vi "DSF.Engine.Memory.ObjectPool.Return Object.vi"(8 "error in (no error)":errorcluster, 9 "timeout ms (0)":i32 format="%d ms", 10 "ObjectPool Bundle":refnum<class "DSF.Engine.Memory.ObjectPool.Bundle.lvclass">, 11 "ObjectPool in":refnum<class "DSF.Engine.Memory.ObjectPool.lvclass">) -> (0 "error out":errorcluster, 1 "timed out?":bool, 3 "ObjectPool out":refnum<class "DSF.Engine.Memory.ObjectPool.lvclass">)   [LabVIEW 2016, in "DSF.Engine.lvlib" / "DSF.Engine.Memory.ObjectPool.lvclass"]
uses:
  DSF.Engine.Memory.ObjectPool.lvclass
  DSF.Engine.Memory.ObjectPool.Bundle.lvclass
  DSF.Engine.Memory.ObjectPool.Bundle.lvclass/DSF.Engine.Memory.ObjectPool.Bundle.ctl
  DSF.Engine.Memory.ObjectPool.lvclass/DSF.Engine.Memory.ObjectPool.ctl
  DSF.Engine.Memory.ObjectPool.Get Index FIFO.vi
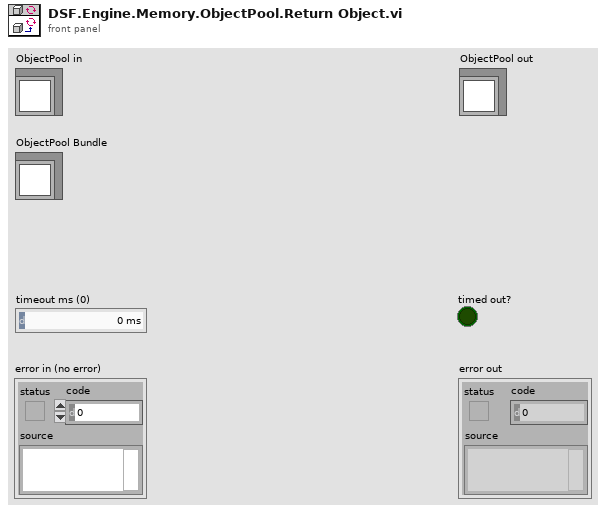
[diagram p1: front panel]
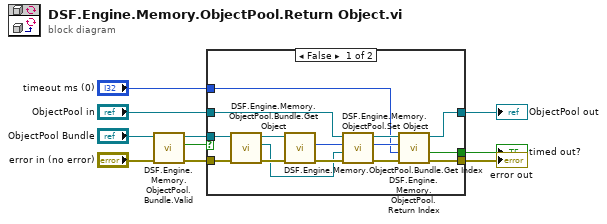
[diagram p0: block diagram]
diagram:
  n1 = call "DSF.Engine.Memory.ObjectPool.Bundle.Valid.vi"("error in (no error)"="error in (no error)", "ObjectPool Bundle in"="ObjectPool Bundle") -> ("error out"=w10:errorcluster, "valid?"=w3:bool, "ObjectPool Bundle out"=w4:refnum<class "DSF.Engine.Memory.ObjectPool.Bundle.lvclass">)  [unwired: 7 in]
  n2 = case shown="False" w3 {
    tunnel: w4 -> [w24 _]
    tunnel: w10 -> [w20 w26]
    tunnel: "ObjectPool in" -> [w19 w25]
    tunnel: [w22 w25] -> w8
    tunnel: [w16 w26] -> w7
    tunnel: "timeout ms (0)" -> [w11 _]
    tunnel: [w12 _] -> w1
    frame False {
      n3 = call "DSF.Engine.Memory.ObjectPool.Bundle.Get Object.vi"("error in (no error)"=w20, "ObjectPool Bundle in"=w24) -> ("error out"=w21:errorcluster, "Object"=w14:refnum<class>, "ObjectPool Bundle out"=w23:refnum<class "DSF.Engine.Memory.ObjectPool.Bundle.lvclass">)  [unwired: 7 in]
      n4 = call "DSF.Engine.Memory.ObjectPool.Bundle.Get Index.vi"("error in (no error)"=w21, "ObjectPool Bundle in"=w23) -> ("error out"=w15:errorcluster, "Index"=w13:i32)  [unwired: 7 in, 1 out]
      n5 = call "DSF.Engine.Memory.ObjectPool.Set Object.vi"("error in (no error)"=w15, "Object"=w14, "index"=w13, "ObjectPool in"=w19) -> ("error out"=w17:errorcluster, "ObjectPool out"=w18:refnum<class "DSF.Engine.Memory.ObjectPool.lvclass">)  [unwired: 6 in]
      n6 = call "DSF.Engine.Memory.ObjectPool.Return Index.vi"("error in (no error)"=w17, "timeout ms (0)"=w11, "index"=w13, "ObjectPool in"=w18) -> ("error out"=w16:errorcluster, "timed out?"=w12:bool, "ObjectPool out"=w22:refnum<class "DSF.Engine.Memory.ObjectPool.lvclass">)  [unwired: 5 in]
    }
    frame True {
      # "#TODO\nThrow error."
    }
  }
  "error out" <- w7
  "ObjectPool out" <- w8
  "timed out?" <- w1
